vi "Add Item.vi"(8 "error in (no error)":errorcluster caption="错误输入（无错误）", 10 "Info":T1={"父项标识符"="", "子项位置"=0, "子项标识符"="", "仅作为子项？"=FALSE, "PicName"="Card.png", "左单元格字符串"=""}, 11 "Tree":refnum<vi>) -> (0 "error out":errorcluster caption="错误输出", 2 "Tag":string, 3 "Tree out":refnum<vi>)   [LabVIEW 2016]
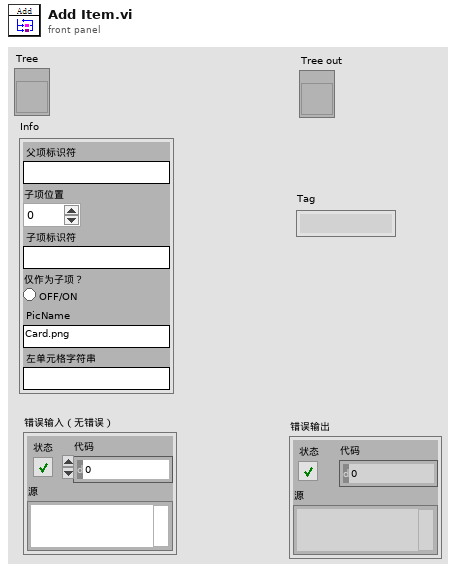
[diagram p1: front panel]
types:
  T1 = cluster{"父项标识符":string, "子项位置":i32, "子项标识符":string, "仅作为子项？":bool, "PicName":string, "左单元格字符串":string}
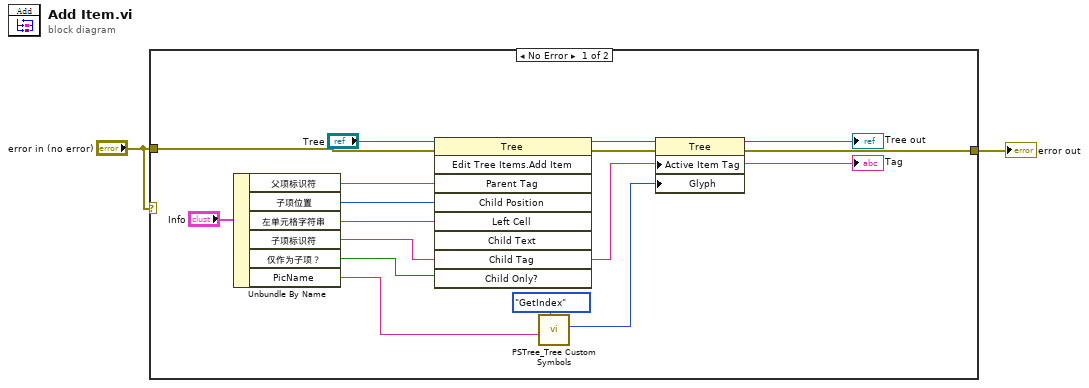
[diagram p0: block diagram]
diagram:
  n1 = case shown="No Error" "error in (no error)" {
    tunnel: [w6 w18] -> w2
    tunnel: "error in (no error)" -> [w5 w18]
    frame No Error {
      n2 = Unbundle By Name("Info") -> ("父项标识符"=w11:string, "子项位置"=w10:i32, "左单元格字符串"=w3:string, "子项标识符"=w4:string, "仅作为子项？"=w9:bool, "PicName"=w8:string)
      "Tag" <- w4
      n3 = invoke class="Tree" method="Edit Tree Items.Add Item"(reference="Tree", error in=w5, "Parent Tag"=w11, "Child Position"=w10, "Left Cell"=w3, "Child Tag"=w4, "Child Only?"=w9) -> (reference out=w16:refnum<vi>, error out=w15:errorcluster)  [unwired: 2 in, 7 out]
      n4 = call "PSTree_Tree Custom Symbols.vi"("Operation"=enum16{"Register", "GetIndex"}."GetIndex", "PicName"=w8) -> ("PicIndex"=w14:i32)  [unwired: 8 in, 1 out]
      n5 = property class="Tree"(reference=w16, error in=w15, "Active Item Tag"=w4, "Glyph"=w14) -> (reference out=→"Tree out":refnum<vi>, error out=w6:errorcluster)
    }
    frame Error {
    }
  }
  "error out" <- w2
